vi "Read_Joint_States.vi"(0 "error in":errorcluster, 2 "Units (deg)":enum16{"Radians", "Degrees"}(ring)=enum."Degrees", 3 "node":string) -> (1 "error out":errorcluster, 4 "Joint States":T1(array[cluster]))   [LabVIEW 2012]
doc: "Read all the current joint states (names, positions, velocity, and efforts)"
uses:
  <userlib>/ROSforLV/ROS/Code/Console/Servers/ServerSubs/TopicDef.ctl
  <userlib>/ROSforLV/ROS/Code/SubVIs/_ROSDirection.ctl
panel:
  out "Reply":string
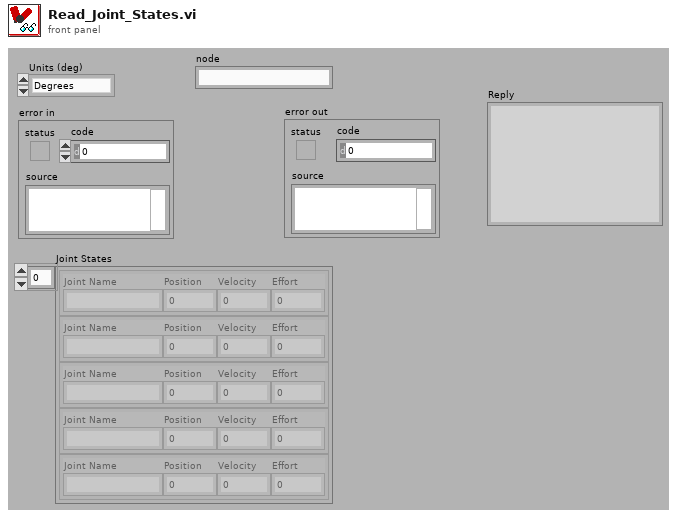
[diagram p1: front panel]
types:
  T1 = cluster{"Joint Name":string, "Position":dbl, "Velocity":dbl, "Effort":dbl}[]
  T2 = typedef "TopicDef.ctl" = cluster{"Topic":string, "Type":string, "Action":T3, "Update (ms)":u16, "write queue":u16}
  T3 = typedef "_ROSDirection.ctl" = enum16{"Node", "Publisher", "Subscriber", "Service Client"}
  T4 = typedef "_ROSControl.ctl" = cluster{"topic port":u16, "Node":string, "topic":string, "type":string, "node port":u16, "error ":errorcluster, "Direction":T3, "APIs":string[], "Update (ms)":u16, "write queue":u16}
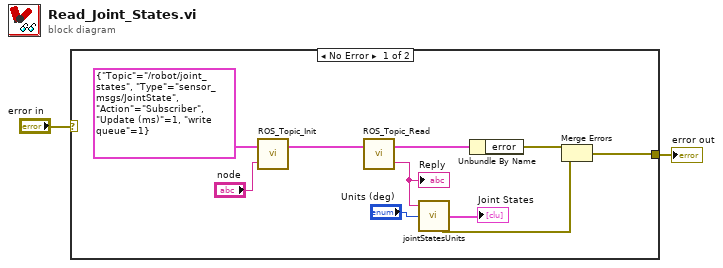
[diagram p0: block diagram]
diagram:
  n1 = case shown="No Error" "error in" {
    selector: "error in" -> [_ w13]
    tunnel: [w3 w13] -> w2
    frame No Error {
      n2 = call <userlib>:"ROS_Topic_Init.vi"("node"="node", "Definitions"=T2 {"Topic"="/robot/joint_states", "Type"="sensor_msgs/JointState", "Action"=enum."Subscriber", "Update (ms)"=1, "write queue"=1}) -> ("ROS out"=w11:T4)  [unwired: 1 in]
      n3 = call <userlib>:"ROS_Topic_Read.vi"("ROS in"=w11) -> ("Reply"=w7:string, "ROS out"=w10:T4)  [unwired: 1 in]
      "Reply" <- w7
      n4 = call <userlib>:"jointStatesUnits.vi"("Units (deg)"="Units (deg)", "msg in"=w7) -> ("error out"=w4:errorcluster, "Joint States"=→"Joint States":T1)  [unwired: 1 in, 1 out]
      n5 = Unbundle By Name(w10) -> ("error"=w5:errorcluster)
      n6 = Merge Errors(w5, w4) -> (w3:errorcluster)
    }
    frame Error {
    }
  }
  "error out" <- w2
